vi "M14_Cowl_Hardware_Globals.vi"() -> ()   [LabVIEW 2019]
panel:
  in  "Cowl Motor":string="Cowl Motor"
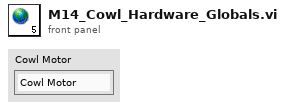
[diagram p1: front panel]
diagram:
